vi "Write ILCAppConfig.vi"(10 "ILCAppConfig":T1={"ILCConfig"={"Input Channels"=enum."Channel 0", "Scan Rate (Hz) "=enum."50", "ADC PGA Gain"=0}, "RS232Config"={"VISA resource name"="", "Baud Rate"=9600, "Data Bits"=8, "Parity"=enum."None", "Stop Bits"=10, "Flow Control"=0, "Timeout (ms)"=10000}, "Application Timing"={"Loop Period (ms)"=1}} {"Application Timing"."Loop Period (ms)" min=1 max=5000; "RS232Config"."Stop Bits" items=["1.0"=10, "1.5"=15, "2.0"=20]; "RS232Config"."Flow Control" items=["None", "XON/XOFF", "RTS/CTS", "XON/XOFF & RTS/CTS", "DTR/DSR", "XON/XOFF & DTR/DSR"]; "RS232Config"."Data Bits" min=5 max=8 step=1; "ILCConfig"."ADC PGA Gain" max=7}, 11 "Start in":refnum<class "Start.lvclass">) -> (3 "Start out":refnum<class "Start.lvclass">)   [LabVIEW 2012, in "Start.lvclass"]
uses:
  Start.lvclass
  State/ILCAppConfig.ctl
  Program Files (x86)/National Instruments/LabVIEW 2012/user.lib/Common/ILC/Configuration/ILCConfig.ctl
  Program Files (x86)/National Instruments/LabVIEW 2012/user.lib/Common/ILC/Configuration/InputChannels.ctl
  Program Files (x86)/National Instruments/LabVIEW 2012/user.lib/Common/ILC/Configuration/ScanRate_Hz_MultichannelOptions.ctl
  Program Files (x86)/National Instruments/LabVIEW 2012/user.lib/Common/SerialProtocols/Configuration/RS232Config.ctl
  Program Files (x86)/National Instruments/LabVIEW 2012/user.lib/Common/Component/Application/Configuration/ApplicationTiming.ctl
  Start.lvclass/Start.ctl
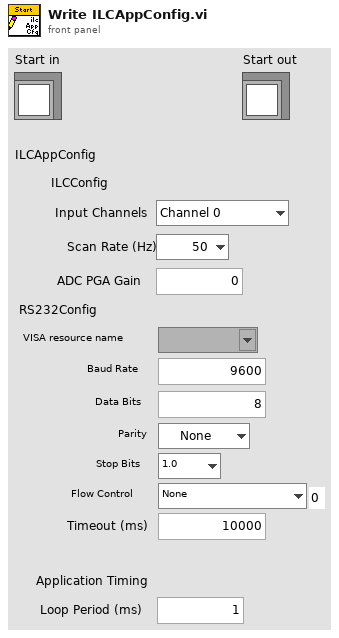
[diagram p1: front panel]
types:
  T1 = typedef "ILCAppConfig.ctl" = cluster{"ILCConfig":T2, "RS232Config":T5, "Application Timing":T6}
  T2 = typedef "ILCConfig.ctl" = cluster{"Input Channels":T3, "Scan Rate (Hz) ":T4, "ADC PGA Gain":u8}
  T3 = typedef "InputChannels.ctl" = enum16{"Channel 0", "3 Channels", "5 Channels"}
  T4 = typedef "ScanRate_Hz_MultichannelOptions.ctl" = enum16{"50", "60", "100", "120", "200", "240", "300", "400", "480", "600", "1200", "2400", "4800"}
  T5 = typedef "RS232Config.ctl" = cluster{"VISA resource name":refnum<visa-resource-name>, "Baud Rate":u32, "Data Bits":u16, "Parity":enum16{"None", "Odd", "Even", "Mark", "Space"}, "Stop Bits":u16, "Flow Control":u16, "Timeout (ms)":u32}
  T6 = typedef "ApplicationTiming.ctl" = cluster{"Loop Period (ms)":u16}
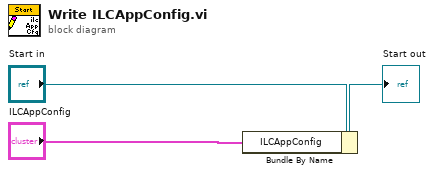
[diagram p0: block diagram]
diagram:
  n1 = Bundle By Name(cluster="Start in", "ILCAppConfig"="ILCAppConfig") -> (→"Start out":refnum<class "Start.lvclass">)
